vi "Intake.vi"(11 "Intake":dbl) -> ()   [LabVIEW 2017]
uses:
  <vilib>/Rock Robotics/WPI/ThirdParty/Phoenix-LabVIEW/Motor Controller/Controls/CTRE_Phoenix_MotorControl_ControlMode.ctl
  <vilib>/Rock Robotics/WPI/ThirdParty/Phoenix-LabVIEW/Motor Controller/Get/CTRE_Phoenix_MotorController_GetVoltage.vi
  <vilib>/Rock Robotics/WPI/ThirdParty/Phoenix-LabVIEW/Motor Controller/Get/CTRE_Phoenix_MotorController_GetOutputCurrent_Enhanced.vi
panel:
  out "Voltage to motors  2":T1(graph)
  out "Voltage to motors":T1(graph)
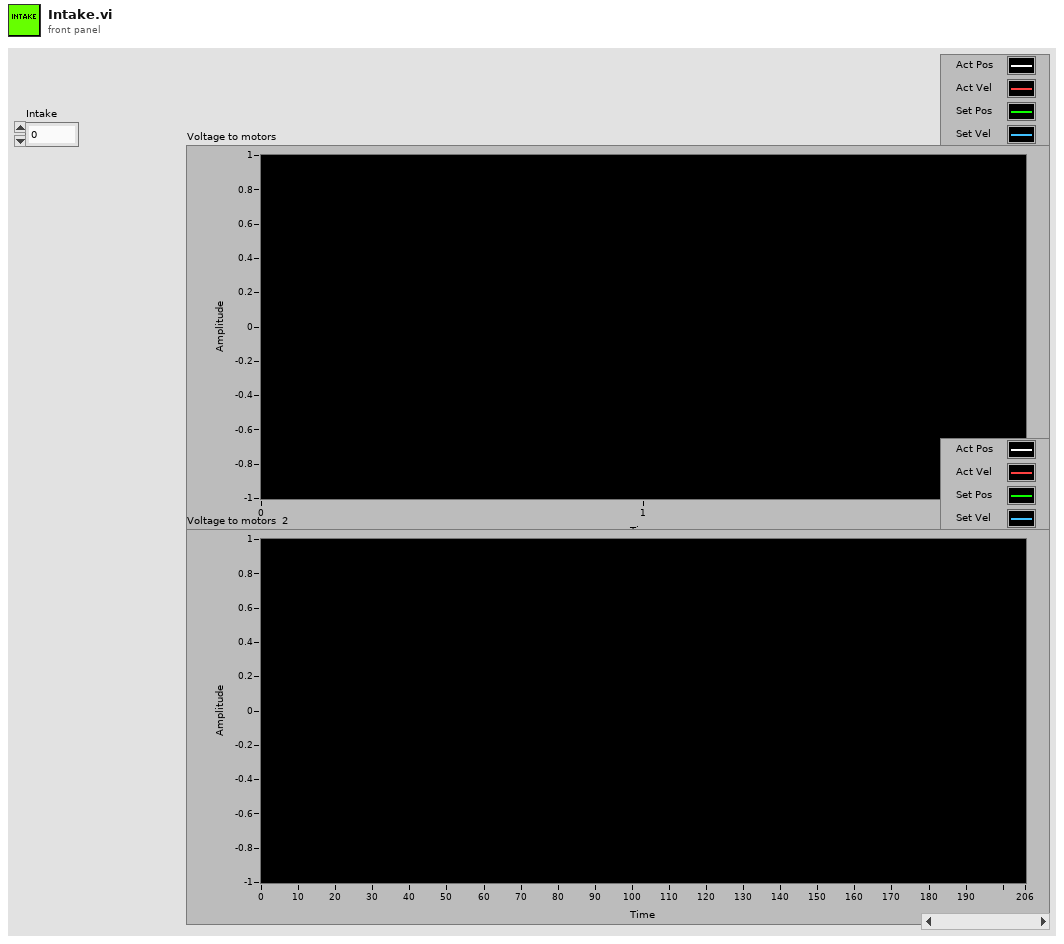
[diagram p1: front panel]
types:
  T1 = cluster{"Percent Output":dbl, "Output Voltage":dbl, "Bus Voltage":dbl, "Output Current":dbl}
  T2 = typedef "CTRE_Phoenix_MotorControl_ControlMode.ctl" = u16
  T3 = typedef "WPI_MotorControlDeviceRef.ctl" = cluster{"DeviceStatus":errorcluster, "Type":T4, "PWM":cluster{"PWM Channel":T5, "DeadBand":T6}, "CAN":cluster{"Device Number":u8, "SetOutput VI Ref":variant, "GetOutput VI Ref":variant, "Enable VI Ref":variant, "Disable VI Ref":variant, "Data":variant}, "Invert":bool, "DIO PWM":cluster{"PWM \"Enable\" Channel":T5, "DIOChannel":T7, "PWM Rate":dbl}}
  T4 = typedef "WPI_MotorControlType.ctl" = enum16{"PWM", "CAN", "DIO PWM"}
  T5 = typedef "FPGA_DIOPWMChannel.ctl" = enum8{"PWM 0", "PWM 1", "PWM 2", "PWM 3", "PWM 4", "PWM 5", "PWM 6", "PWM 7", "PWM 8", "PWM 9", "PWM MXP 0", "PWM MXP 1", "PWM MXP 2", "PWM MXP 3", "PWM MXP 4", "PWM MXP 5", "PWM MXP 6", "PWM MXP 7", "PWM MXP 8", "PWM MXP 9", "Invalid"}
  T6 = typedef "WPI_PWMDeadband.ctl" = cluster{"Name":string, "maxPositivePwm":i32, "minPositivePwm":i32, "centerPwm":i32, "maxNegativePwm":i32, "minNegativePwm":i32, "angularRange":u16}
  T7 = typedef "FPGA_DIOChannel.ctl" = enum8{"DIO 0", "DIO 1", "DIO 2", "DIO 3", "DIO 4", "DIO 5", "DIO 6", "DIO 7", "DIO 8", "DIO 9", "DIO MXP 0", "DIO MXP 1", "DIO MXP 2", "DIO MXP 3", "DIO MXP 4", "DIO MXP 5", "DIO MXP 6", "DIO MXP 7", "DIO MXP 8", "DIO MXP 9", "DIO MXP 10", "DIO MXP 11", "DIO MXP 12", "DIO MXP 13", "DIO MXP 14", "DIO MXP 15", "SPI Port CS1", "SPI Port CS2", "SPI Port CS3", "SPI Port MISO", "SPI Port MOSI", "Invalid"}
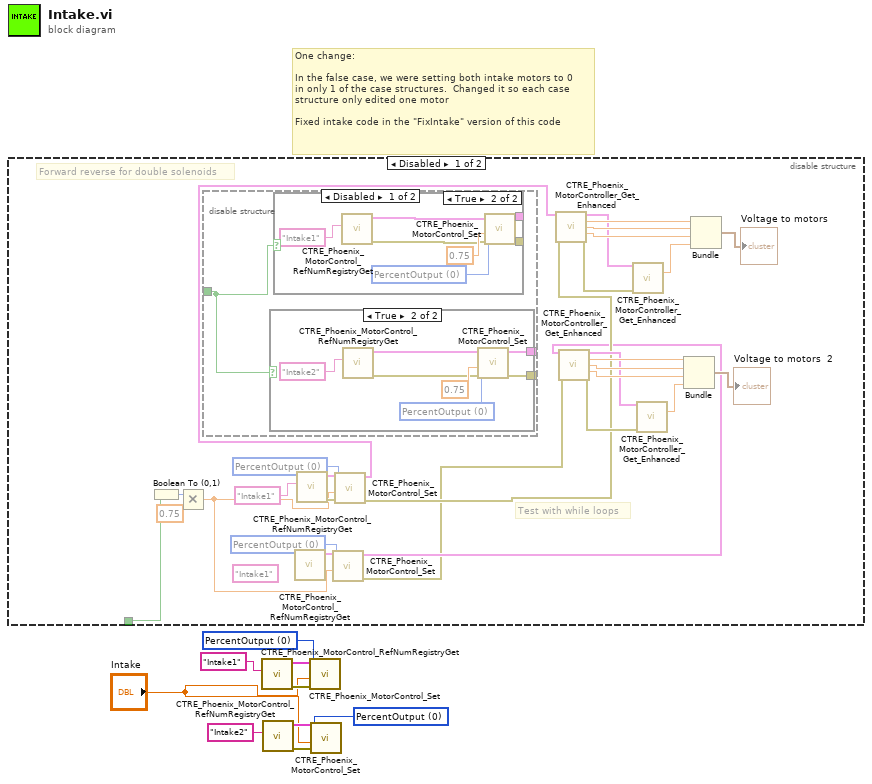
[diagram p0: block diagram]
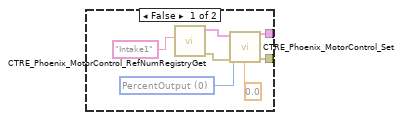
[diagram p2: hidden frame]
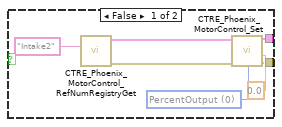
[diagram p3: hidden frame]
diagram:
  w3 = T2 0 items=["PercentOutput"=0, "Position"=1, "Velocity"=2, "Current"=3, "Follower"=5, "MotionProfile"=6, "MotionMagic"=7, "MotionMagicArc"=8, "MotionProfileArc"=10, "Disabled"=15] ("Control Mode")
  w6 = T2 0 items=["PercentOutput"=0, "Position"=1, "Velocity"=2, "Current"=3, "Follower"=5, "MotionProfile"=6, "MotionMagic"=7, "MotionMagicArc"=8, "MotionProfileArc"=10, "Disabled"=15] ("Control Mode")
  # "One change: \n\nIn the false case, we were setting both intake motors to 0\nin only 1 of the case structures.  Changed it so each case\nstructure only edited one motor\n\nFixed intake code in the \"FixIntake\" version of this code"
  n1 = disable-structure shown="Disabled" {
    disable-tunnel: _ -> [w10 _]
    frame Disabled {
      w17 = T2 0 items=["PercentOutput"=0, "Position"=1, "Velocity"=2, "Current"=3, "Follower"=5, "MotionProfile"=6, "MotionMagic"=7, "MotionMagicArc"=8, "MotionProfileArc"=10, "Disabled"=15] ("Control Mode")
      (unwired) "Intake1" ("refnum name")
      w20 = T2 0 items=["PercentOutput"=0, "Position"=1, "Velocity"=2, "Current"=3, "Follower"=5, "MotionProfile"=6, "MotionMagic"=7, "MotionMagicArc"=8, "MotionProfileArc"=10, "Disabled"=15] ("Control Mode")
      # "Test with while loops"
      # "Forward reverse for double solenoids"
      n2 = Boolean To (0,1)(Boolean=w10) -> (0, 1=w19:i16)
      n3 = Multiply(x=w19, y=0.75) -> (x*y=w15:dbl)
      n4 = disable-structure shown="Disabled" {
        disable-tunnel: [w40 _] -> _
        disable-tunnel: [w39 _] -> _
        disable-tunnel: _ -> [w38 _]
        frame Disabled {
          n5 = case shown="True" w38 {
            tunnel: [w58 w65] -> w40
            tunnel: [w57 w64] -> w39
            frame False {
              w60 = T2 0 items=["PercentOutput"=0, "Position"=1, "Velocity"=2, "Current"=3, "Follower"=5, "MotionProfile"=6, "MotionMagic"=7, "MotionMagicArc"=8, "MotionProfileArc"=10, "Disabled"=15] ("Control Mode")
              n6 = call <vilib>:"CTRE_Phoenix_MotorControl_RefNumRegistryGet.vi"("refnum name"="Intake2") -> ("error out"=w55:errorcluster, "PhoenixMotorControlDevRef"=w56:T3)  [unwired: 9 in]
              n7 = call <vilib>:"CTRE_Phoenix_MotorControl_Set.vi"("error in (no error)"=w55, "Output"=0.0, "Control Mode"=w60, "PhoenixMotorControlDevRef"=w56) -> ("error out"=w57:errorcluster, "PhoenixMotorControlDevRef"=w58:T3)  [unwired: 6 in]
            }
            frame True {
              w66 = T2 0 items=["PercentOutput"=0, "Position"=1, "Velocity"=2, "Current"=3, "Follower"=5, "MotionProfile"=6, "MotionMagic"=7, "MotionMagicArc"=8, "MotionProfileArc"=10, "Disabled"=15] ("Control Mode")
              n8 = call <vilib>:"CTRE_Phoenix_MotorControl_RefNumRegistryGet.vi"("refnum name"="Intake2") -> ("error out"=w62:errorcluster, "PhoenixMotorControlDevRef"=w63:T3)  [unwired: 9 in]
              n9 = call <vilib>:"CTRE_Phoenix_MotorControl_Set.vi"("error in (no error)"=w62, "Output"=0.75, "Control Mode"=w66, "PhoenixMotorControlDevRef"=w63) -> ("error out"=w64:errorcluster, "PhoenixMotorControlDevRef"=w65:T3)  [unwired: 6 in]
            }
          }
          n10 = case shown="True" w38 {
            tunnel: [w43 w51] -> _
            tunnel: [w42 w50] -> _
            frame False {
              w44 = T2 0 items=["PercentOutput"=0, "Position"=1, "Velocity"=2, "Current"=3, "Follower"=5, "MotionProfile"=6, "MotionMagic"=7, "MotionMagicArc"=8, "MotionProfileArc"=10, "Disabled"=15] ("Control Mode")
              n11 = call <vilib>:"CTRE_Phoenix_MotorControl_RefNumRegistryGet.vi"("refnum name"="Intake1") -> ("error out"=w41:errorcluster, "PhoenixMotorControlDevRef"=w47:T3)  [unwired: 9 in]
              n12 = call <vilib>:"CTRE_Phoenix_MotorControl_Set.vi"("error in (no error)"=w41, "Output"=0.0, "Control Mode"=w44, "PhoenixMotorControlDevRef"=w47) -> ("error out"=w42:errorcluster, "PhoenixMotorControlDevRef"=w43:T3)  [unwired: 6 in]
            }
            frame True {
              w52 = T2 0 items=["PercentOutput"=0, "Position"=1, "Velocity"=2, "Current"=3, "Follower"=5, "MotionProfile"=6, "MotionMagic"=7, "MotionMagicArc"=8, "MotionProfileArc"=10, "Disabled"=15] ("Control Mode")
              n13 = call <vilib>:"CTRE_Phoenix_MotorControl_RefNumRegistryGet.vi"("refnum name"="Intake1") -> ("error out"=w48:errorcluster, "PhoenixMotorControlDevRef"=w49:T3)  [unwired: 9 in]
              n14 = call <vilib>:"CTRE_Phoenix_MotorControl_Set.vi"("error in (no error)"=w48, "Output"=0.75, "Control Mode"=w52, "PhoenixMotorControlDevRef"=w49) -> ("error out"=w50:errorcluster, "PhoenixMotorControlDevRef"=w51:T3)  [unwired: 6 in]
            }
          }
        }
        frame Enabled {
        }
      }
      n15 = call <vilib>:"CTRE_Phoenix_MotorControl_RefNumRegistryGet.vi"() -> ("PhoenixMotorControlDevRef"=w16:T3)  [unwired: 10 in, 1 out]
      n16 = call <vilib>:"CTRE_Phoenix_MotorControl_RefNumRegistryGet.vi"("refnum name"="Intake1") -> ("error out"=w21:errorcluster, "PhoenixMotorControlDevRef"=w22:T3)  [unwired: 9 in]
      n17 = call <vilib>:"CTRE_Phoenix_MotorControl_Set.vi"("Output"=w15, "Control Mode"=w17, "PhoenixMotorControlDevRef"=w16) -> ("error out"=w11:errorcluster, "PhoenixMotorControlDevRef"=w12:T3)  [unwired: 7 in]
      n18 = call <vilib>:"CTRE_Phoenix_MotorControl_Set.vi"("error in (no error)"=w21, "Output"=w15, "Control Mode"=w20, "PhoenixMotorControlDevRef"=w22) -> ("error out"=w13:errorcluster, "PhoenixMotorControlDevRef"=w14:T3)  [unwired: 6 in]
      n19 = call-poly <vilib>:"CTRE_Phoenix_MotorController_Get_Enhanced.vi"("PhoenixMotorControlDevRef"=w14, "error in"=w13) -> ("PhoenixMotorControlDevRef"=w25:T3, "Percent Output"=w37:dbl, "Output Voltage"=w36:dbl, "Bus Voltage"=w35:dbl, "error out"=w24:errorcluster)  [unwired: 9 in]
      n20 = call-poly <vilib>:"CTRE_Phoenix_MotorController_Get_Enhanced.vi"("PhoenixMotorControlDevRef"=w12, "error in"=w11) -> ("PhoenixMotorControlDevRef"=w27:T3, "Percent Output"=w30:dbl, "Output Voltage"=w31:dbl, "Bus Voltage"=w32:dbl, "error out"=w26:errorcluster)  [unwired: 9 in]
      n21 = call-poly <vilib>:"CTRE_Phoenix_MotorController_Get_Enhanced.vi"("PhoenixMotorControlDevRef"=w25, "error in"=w24) -> ("Output Current"=w29:dbl)  [unwired: 11 in, 2 out]
      n22 = call-poly <vilib>:"CTRE_Phoenix_MotorController_Get_Enhanced.vi"("PhoenixMotorControlDevRef"=w27, "error in"=w26) -> ("Output Current"=w28:dbl)  [unwired: 11 in, 2 out]
      n23 = Bundle("Percent Output"=w30, "Output Voltage"=w31, "Bus Voltage"=w32, "Output Current"=w28) -> (→"Voltage to motors  2":T1)  [unwired: 1 in]
      n24 = Bundle("Percent Output"=w37, "Output Voltage"=w36, "Bus Voltage"=w35, "Output Current"=w29) -> (→"Voltage to motors":T1)  [unwired: 1 in]
    }
    frame Enabled {
    }
  }
  n25 = call <vilib>:"CTRE_Phoenix_MotorControl_RefNumRegistryGet.vi"("refnum name"="Intake1") -> ("error out"=w7:errorcluster, "PhoenixMotorControlDevRef"=w8:T3)  [unwired: 9 in]
  n26 = call <vilib>:"CTRE_Phoenix_MotorControl_RefNumRegistryGet.vi"("refnum name"="Intake2") -> ("error out"=w4:errorcluster, "PhoenixMotorControlDevRef"=w5:T3)  [unwired: 9 in]
  n27 = call <vilib>:"CTRE_Phoenix_MotorControl_Set.vi"("error in (no error)"=w7, "Output"="Intake", "Control Mode"=w6, "PhoenixMotorControlDevRef"=w8) -> ()  [unwired: 6 in, 2 out]
  n28 = call <vilib>:"CTRE_Phoenix_MotorControl_Set.vi"("error in (no error)"=w4, "Output"="Intake", "Control Mode"=w3, "PhoenixMotorControlDevRef"=w5) -> ()  [unwired: 6 in, 2 out]
